vi "Find NI-SWITCH Custom Device.vi"   [LabVIEW 2017, in "NI-SWITCH Scripting.lvlib"]
uses:
  NI-SWITCH Scripting.lvlib
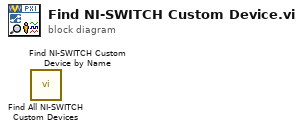
[diagram p0: block diagram]
diagram:
  n1 = call "Find All NI-SWITCH Custom Devices.vi"() -> ()  [unwired: 9 in, 3 out]
  n2 = call "Find NI-SWITCH Custom Device by Name.vi"() -> ()  [unwired: 9 in, 3 out]
